vi "Start.vi"(8 "error in (no error)":errorcluster, 10 "ASync [T]":bool, 11 "iService in":refnum<class "iService.lvclass">) -> (0 "error out":errorcluster, 3 "iService out":refnum<class "iService.lvclass">)   [LabVIEW 2019, in "gRPC-servicer.lvlib" / "iService.lvclass"]
uses:
  iService.lvclass
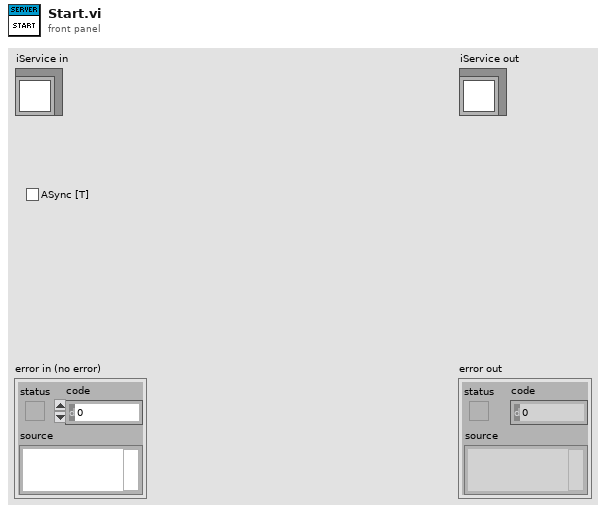
[diagram p1: front panel]
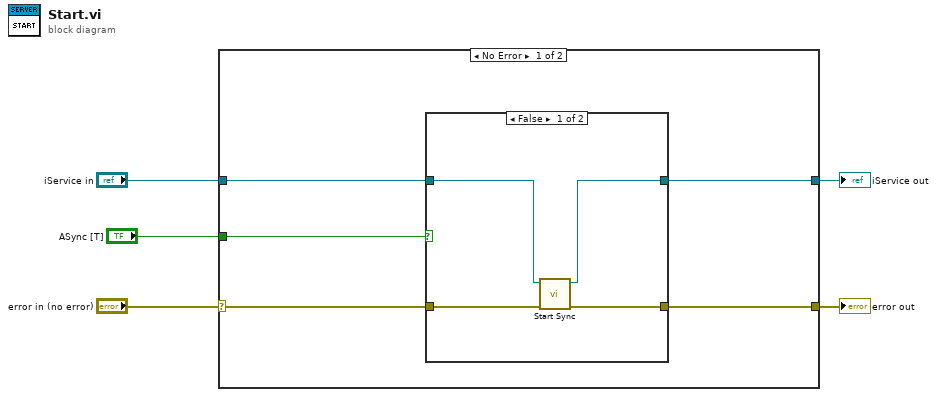
[diagram p0: block diagram]
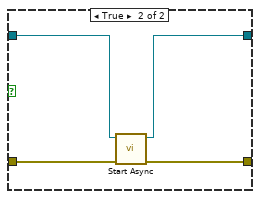
[diagram p2: hidden frame]
diagram:
  n1 = case shown="No Error" "error in (no error)" {
    selector: "error in (no error)" -> [w10 w20]
    tunnel: [w9 w20] -> w4
    tunnel: [w7 w19] -> w2
    tunnel: "iService in" -> [w8 w19]
    tunnel: "ASync [T]" -> [w6 _]
    frame No Error {
      n2 = case shown="False" w6 {
        tunnel: w10 -> [w14 w18]
        tunnel: [w13 w17] -> w9
        tunnel: w8 -> [w12 w16]
        tunnel: [w11 w15] -> w7
        frame False {
          n3 = call-dynamic "Start Sync.vi"("error in (no error)"=w14, "gRPC Server in"=w12) -> ("error out"=w13:errorcluster, "gRPC Server out"=w11:refnum<class "iService.lvclass">)  [unwired: 8 in]
        }
        frame True {
          n4 = call-dynamic "Start Async.vi"("error in (no error)"=w18, "gRPC Server in"=w16) -> ("error out"=w17:errorcluster, "gRPC Server out"=w15:refnum<class "iService.lvclass">)  [unwired: 8 in]
        }
      }
    }
    frame Error {
    }
  }
  "error out" <- w4
  "iService out" <- w2
